vi "ManagerEventClose.vi"(8 "error in (no error)":errorcluster, 10 "Event Registration Refnum In":refnum<event-registration>, 11 "Manager In":u64 caption="Device In") -> (0 "error out":errorcluster, 3 "Manager Out":u64 caption="Device Out")   [LabVIEW 2012, in "Phidget Manager.lvlib"]
doc: "${AccelerationChange:CloseHeader}"
uses:
  <instrlib>/Phidgets/Phidget Manager/Phidget Manager.lvlib
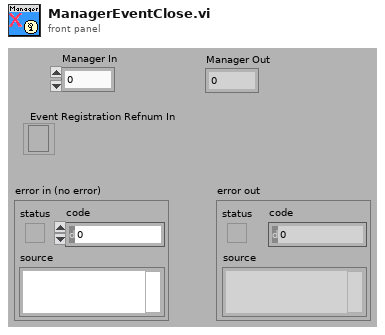
[diagram p1: front panel]
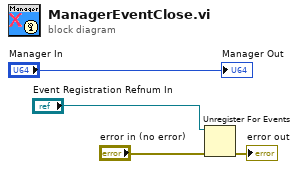
[diagram p0: block diagram]
diagram:
  n1 = Unregister For Events(event registration refnum="Event Registration Refnum In", error in="error in (no error)") -> (error out=→"error out":errorcluster)
  "Manager Out" <- "Manager In"
